vi "T Vector Filter.vi"(9 "Tag ID":i32, 10 "t Translation Vector":dbl[](array[numeric]) format="%#.6f") -> (2 "t Translation Vector filtered":dbl[](array[numeric]))   [LabVIEW 2025]
panel:
  out "Filtered Data":dbl[][](array[numeric])
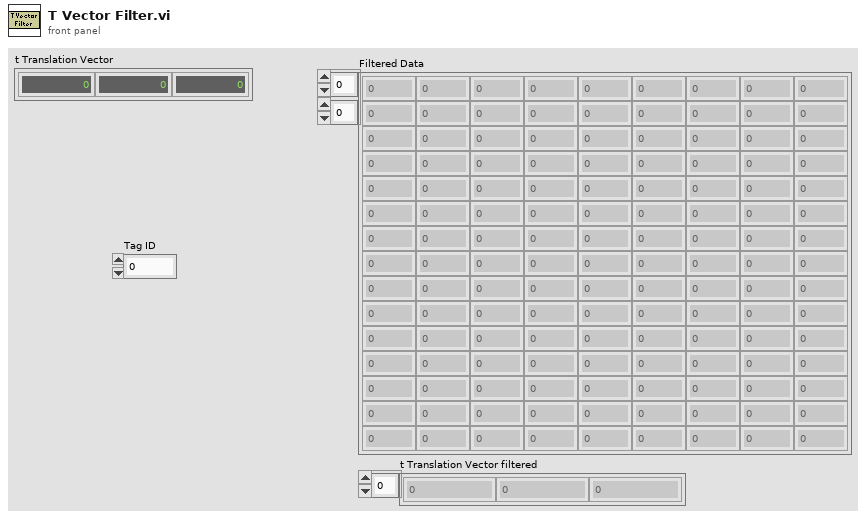
[diagram p1: front panel]
types:
  T1 = cluster{"Previous Position ":dbl[][], "Filter Factor a":dbl[], "Velocity Previous":dbl[][], "Filter Factor ß":dbl[]}
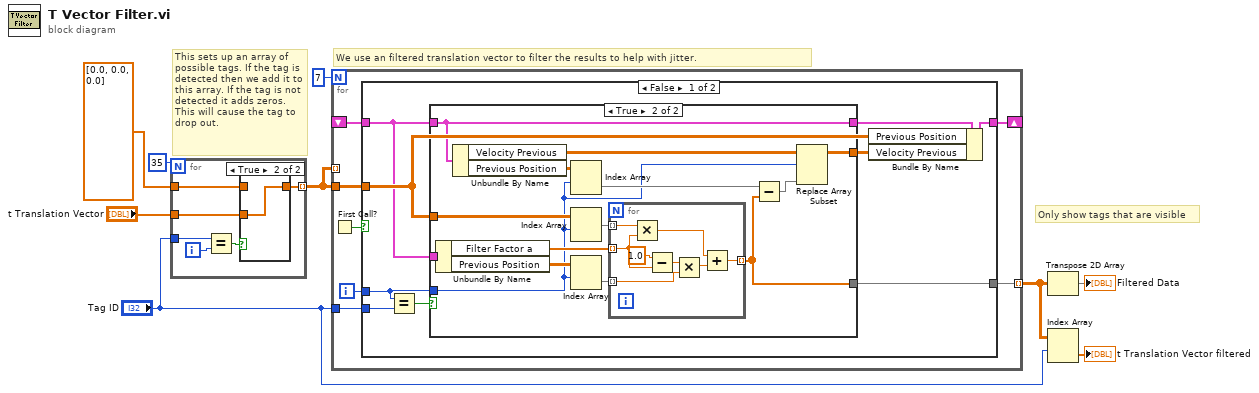
[diagram p0: block diagram]
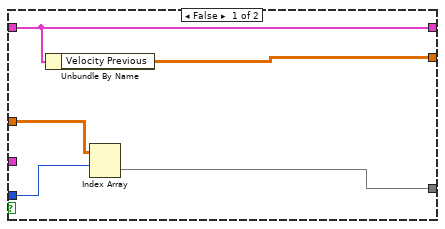
[diagram p2: hidden frame]
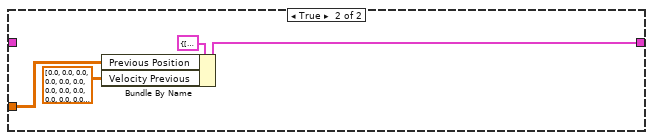
[diagram p3: hidden frame]
diagram:
  # "Only show tags that are visible"
  # "We use an filtered translation vector to filter the results to help with jitter."
  # "This sets up an array of possible tags. If the tag is detected then we add it to this array. If the tag is not detected it adds zeros. This will cause the tag to drop out."
  n1 = for {
    N: 35 -> [_]
    tunnel: dbl[] [0.0, 0.0, 0.0] ("f") -> [w15]
    tunnel: "t Translation Vector" -> [w10]
    tunnel: [w14] -> w6 mode=indexing
    tunnel: "Tag ID" -> [w12]
    i -> [w13]
    n2 = Equal?(x=w12, y=w13) -> (x = y?=w11:bool)
    n3 = case shown="True" w11 {
      tunnel: w10 -> [_ w17]
      tunnel: [w16 w17] -> w14
      tunnel: w15 -> [w16 _]
      frame False {
      }
      frame True {
      }
    }
  }
  n4 = for {
    N: 7 -> [_]
    shift-right: [w24] -> _
    shift-left: _ -> [w22]
    tunnel: [w21] -> w1 mode=indexing
    tunnel: w6 -> [w23]
    tunnel: "Tag ID" -> [w19]
    tunnel: w6 -> [_] mode=indexing
    i -> [w20]
    n5 = First Call?() -> (First Call?: T/F=w18:bool)
    n6 = case shown="False" w18 {
      tunnel: [w33 w64] -> w24
      tunnel: w23 -> [w32 w63]
      tunnel: w22 -> [w25 _]
      tunnel: [w29 _] -> w21
      tunnel: w20 -> [w27 _]
      tunnel: w19 -> [w26 _]
      frame False {
        n7 = Equal?(x=w27, y=w26) -> (x = y?=w28:bool)
        n8 = case shown="True" w28 {
          tunnel: w32 -> [w38 w50]
          tunnel: w25 -> [_ w52]
          tunnel: [w36 w43] -> w29
          tunnel: w27 -> [w37 w40]
          tunnel: w25 -> [w35 w46]
          tunnel: [w35 w46] -> w31
          tunnel: [w34 w41] -> w30
          frame False {
            n9 = Unbundle By Name(w35) -> ("Velocity Previous"=w34:dbl[][])
            n10 = Index Array(array=w38, index (row)=w37) -> (element=w36:dbl[])  [unwired: 1 in]
          }
          frame True {
            n11 = Unbundle By Name(w52) -> ("Filter Factor a"=w51:dbl[], "Previous Position"=w48:dbl[][])
            n12 = Unbundle By Name(w46) -> ("Velocity Previous"=w42:dbl[][], "Previous Position"=w45:dbl[][])
            n13 = Index Array(array=w45, index (row)=w40) -> (element=w44:dbl[])  [unwired: 1 in]
            n14 = Index Array(array=w50, index (row)=w40) -> (element=w49:dbl[])  [unwired: 1 in]
            n15 = Index Array(array=w48, index (row)=w40) -> (element=w47:dbl[])  [unwired: 1 in]
            n16 = for {
              tunnel: w51 -> [w54] mode=indexing
              tunnel: w49 -> [w53] mode=indexing
              tunnel: w47 -> [w56] mode=indexing
              tunnel: [w55] -> w43 mode=indexing
              n17 = Multiply(x=w53, y=w54) -> (x*y=w57:dbl)
              n18 = Subtract(x=1.0, y=w54) -> (x-y=w59:dbl)
              n19 = Multiply(x=w59, y=w56) -> (x*y=w58:dbl)
              n20 = Add(x=w57, y=w58) -> (x+y=w55:dbl)
            }
            n21 = Subtract(x=w44, y=w43) -> (x-y=w39:dbl[])
            n22 = Replace Array Subset(array=w42, new element=w39, index (row)=w40) -> (w41:dbl[][])  [unwired: 1 in]
          }
        }
        n23 = Bundle By Name(cluster=w31, "Previous Position"=w32, "Velocity Previous"=w30) -> (w33:T1)
      }
      frame True {
        n24 = Bundle By Name(cluster=T1 {"Previous Position "=[], "Filter Factor a"=[0.25, 0.25, 0.2], "Velocity Previous"=[], "Filter Factor ß"=[0.1, 0.1, 0.1]}, "Previous Position"=w63, "Velocity Previous"=dbl[][] [[0.0, 0.0, 0.0, 0.0], [0.0, 0.0, 0.0, 0.0], [0.0, 0.0, 0.0, 0.0], [0.0, 0.0, 0.0, 0.0], [0.0, 0.0, 0.0, 0.0], [0.0, 0.0, 0.0, 0.0], [0.0, 0.0, 0.0, 0.0], [0.0, 0.0, 0.0, 0.0], [0.0, 0.0, 0.0, 0.0], [0.0, 0.0, 0.0, 0.0], [0.0, 0.0, 0.0, 0.0], [0.0, 0.0, 0.0, 0.0], [0.0, 0.0, 0.0, 0.0], [0.0, 0.0, 0.0, 0.0], [0.0, 0.0, 0.0, 0.0], [0.0, 0.0, 0.0, 0.0], [0.0, 0.0, 0.0, 0.0], [0.0, 0.0, 0.0, 0.0], [0.0, 0.0, 0.0, 0.0], [0.0, 0.0, 0.0, 0.0], [0.0, 0.0, 0.0, 0.0], [0.0, 0.0, 0.0, 0.0], [0.0, 0.0, 0.0, 0.0], [0.0, 0.0, 0.0, 0.0], [0.0, 0.0, 0.0, 0.0], [0.0, 0.0, 0.0, 0.0], [0.0, 0.0, 0.0, 0.0], [0.0, 0.0, 0.0, 0.0], [0.0, 0.0, 0.0, 0.0], [0.0, 0.0, 0.0, 0.0], [0.0, 0.0, 0.0, 0.0], [0.0, 0.0, 0.0, 0.0], [0.0, 0.0, 0.0, 0.0], [0.0, 0.0, 0.0, 0.0], [0.0, 0.0, 0.0, 0.0], [0.0, 0.0, 0.0, 0.0]]) -> (w64:T1)
      }
    }
  }
  n25 = Transpose 2D Array(2D array=w1) -> (transposed array=→"Filtered Data":dbl[][])
  n26 = Index Array(array=w1, index (row)="Tag ID") -> (element=→"t Translation Vector filtered":dbl[])  [unwired: 1 in]
